vi "ELVIS III v1.0 Close AO Block.vi"(8 "error in (no error)":errorcluster, 10 "AO (N Samples) Channel List":T3, 11 "myRIO Ref In":T1) -> (0 "error out":errorcluster)   [LabVIEW 2021]
uses:
  <vilib>/myRIO/Common/Instrument Driver Framework/myRIO v1.0/AO Block/typedefs/AO Block Channels List.ctl
  <vilib>/myRIO/Common/Instrument Driver Framework/myRIO v1.0/AO Block/typedefs/AO Block Channels Enum.ctl
  <vilib>/myRIO/Common/Instrument Driver Framework/Utilities/typedefs/myRIO v1.0 Reference.ctl
  <vilib>/myRIO/Common/Instrument Driver Framework/Utilities/typedefs/Generic FPGA Reference.ctl
  <vilib>/myRIO/Common/Instrument Driver Framework/ELVIS III v1.0/AO Block/vis/ELVIS III v1.0 Build MUX Configuration AO Block.vi
  <vilib>/myRIO/Common/Instrument Driver Framework/ELVIS III v1.0/Resource Manager/vis/ELVIS III v1.0 Unreserve Channel List.vi
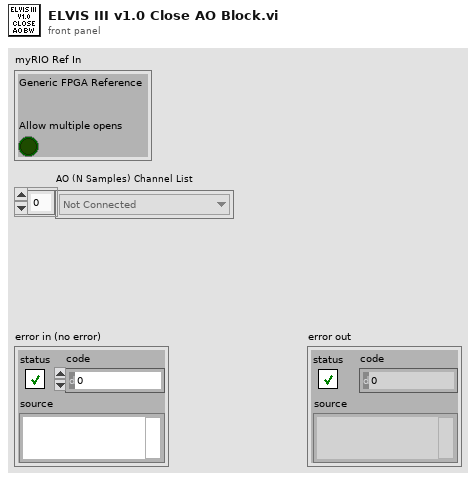
[diagram p1: front panel]
types:
  T1 = typedef "myRIO v1.0 Reference.ctl" = cluster{"Generic FPGA Reference":T2, "Allow multiple opens":bool}
  T2 = typedef "Generic FPGA Reference.ctl" = refnum<k20>
  T3 = typedef "AO Block Channels List.ctl" = T4[]
  T4 = typedef "AO Block Channels Enum.ctl" = enum16{"Not Connected", "A/AO0 (N Samples)", "A/AO1 (N Samples)", "B/AO0 (N Samples)", "B/AO1 (N Samples)"}
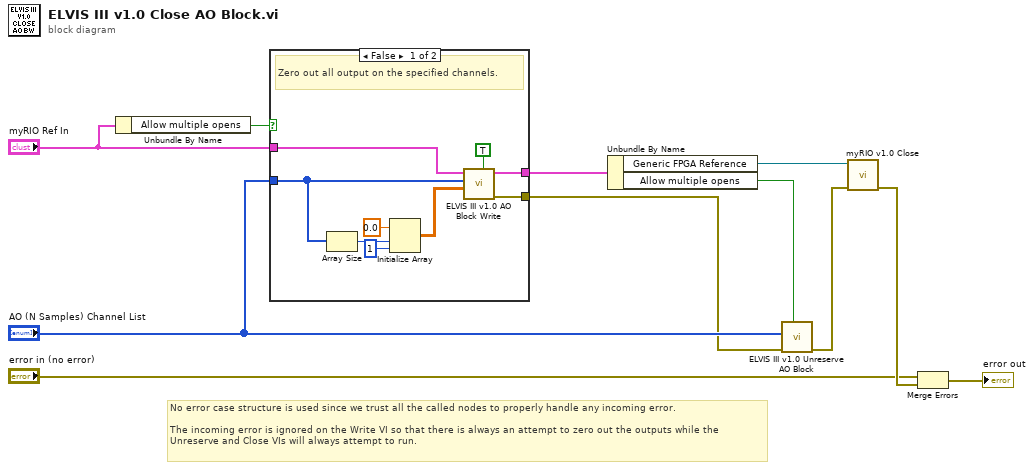
[diagram p0: block diagram]
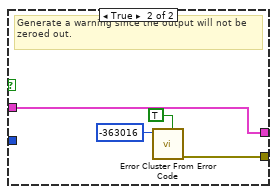
[diagram p2: hidden frame]
diagram:
  # "No error case structure is used since we trust all the called nodes to properly handle any incoming error.\n\nThe incoming error is ignored on the Write VI so that there is always an attempt to zero out the outputs while the Unreserve and Close VIs will always attempt to run."
  n1 = Unbundle By Name("myRIO Ref In") -> ("Allow multiple opens"=w6:bool)
  n2 = case shown="False" w6 {
    tunnel: "AO (N Samples) Channel List" -> [w17 _]
    tunnel: "myRIO Ref In" -> [w19 w23]
    tunnel: [w13 w23] -> w10
    tunnel: [w12 w24] -> w1
    frame False {
      # "Zero out all output on the specified channels."
      n3 = Array Size(array=w17) -> (size(s)=w15:i32)
      n4 = Initialize Array(0.0 ("element"), w15, 1 ("dimension size")) -> (w20:dbl[][])
      n5 = call <vilib>:"ELVIS III v1.0 AO Block Write.vi"("Wait Until Done?"=TRUE, "dbl Scaled Value List"=w20, "AO (N Samples) Channel List"=w17, "myRIO Ref In"=w19) -> ("error out"=w12:errorcluster, "myRIO Ref Out"=w13:T1)  [unwired: 6 in]
    }
    frame True {
      # "Generate a warning since the output will not be zeroed out."
      n6 = call <vilib>:"Error Cluster From Error Code.vi"("is warning? (False)"=TRUE, "error code (0)"=-363016) -> ("error out"=w24:errorcluster)  [unwired: 7 in]
    }
  }
  n7 = Unbundle By Name(w10) -> ("Generic FPGA Reference"=w3:T2, "Allow multiple opens"=w5:bool)
  n8 = call <vilib>:"ELVIS III v1.0 Unreserve AO Block.vi"("Allow multiple opens?"=w5, "error in (no error)"=w1, "AO (N Samples) Channel List"="AO (N Samples) Channel List") -> ("error out"=w9:errorcluster)  [unwired: 8 in]
  n9 = call <vilib>:"myRIO v1.0 Close.vi"("error in (no error)"=w9, "myRIO FPGA Ref In"=w3) -> ("error out"=w8:errorcluster)  [unwired: 9 in]
  n10 = Merge Errors("error in (no error)", w8) -> (→"error out":errorcluster)
